vi "Prober_ChuckStatusCheck.vi"(8 "error in (no error)":errorcluster, 11 "ProbeStationControl in":refnum<class "ProbeStationControl.lvclass">) -> (0 "error out":errorcluster, 2 "Chuck at CONTACT?":bool=TRUE, 3 "ProbeStationControl out":refnum<class "ProbeStationControl.lvclass">)   [LabVIEW 2018, in "ProbeStationControl.lvclass"]
uses:
  ProbeStationControl.lvclass
  ProbeStationControl.lvclass/ProbeStationControl.ctl
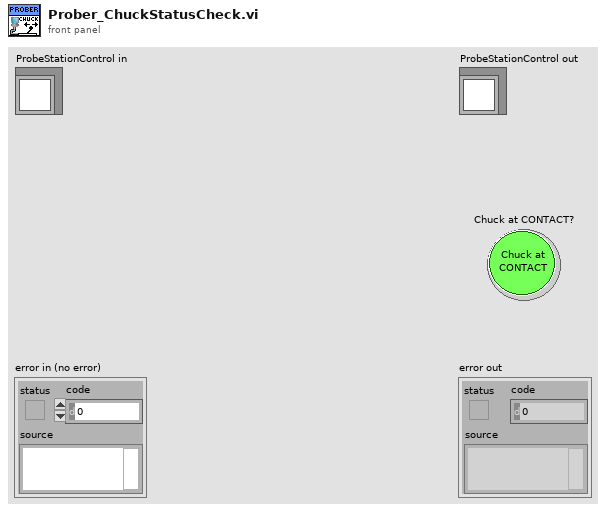
[diagram p1: front panel]
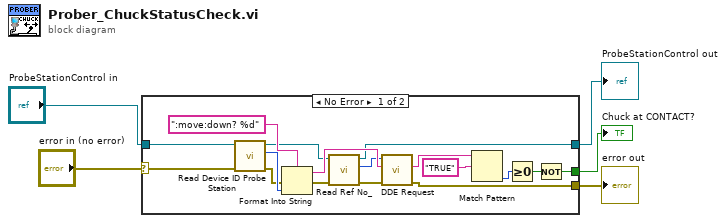
[diagram p0: block diagram]
diagram:
  n1 = case shown="No Error" "error in (no error)" {
    selector: "error in (no error)" -> [w8 w24]
    tunnel: [w12 w24] -> w4
    tunnel: "ProbeStationControl in" -> [w10 w23]
    tunnel: [w7 _] -> w2
    tunnel: [w6 w23] -> w1
    frame No Error {
      n2 = call "Read Device ID Probe Station.vi"("error in (no error)"=w8, "ProbeStationControl in"=w10) -> ("error out"=w15:errorcluster, "Device ID Probe Station"=w16:u32, "ProbeStationControl out"=w9:refnum<class "ProbeStationControl.lvclass">)  [unwired: 7 in]
      n3 = Format Into String(format string=":move:down? %d" ("item"), error in=w15, w16) -> (resulting string=w17:string, error out=w14:errorcluster)  [unwired: 1 in]
      n4 = call "Read Ref No_.vi"("error in (no error)"=w14, "ProbeStationControl in"=w9) -> ("error out"=w13:errorcluster, "Ref No."=w11:i32, "ProbeStationControl out"=w6:refnum<class "ProbeStationControl.lvclass">)  [unwired: 7 in]
      n5 = call <vilib>:"DDE Request.vi"("error in (no error)"=w13, "item"=w17, "conversation refnum in"=w11) -> ("error out"=w12:errorcluster, "data"=w20:string)  [unwired: 4 in, 1 out]
      n6 = Match Pattern(string=w20, regular expression="TRUE") -> (offset past match=w22:i32)  [unwired: 1 in, 3 out]
      n7 = Greater Or Equal To 0?(x=w22) -> (x >= 0?=w19:bool)
      n8 = Not(x=w19) -> (.not. x?=w7:bool)
    }
    frame Error {
    }
  }
  "error out" <- w4
  "Chuck at CONTACT?" <- w2
  "ProbeStationControl out" <- w1
